vi "logging_stop.vi"(8 "error in":errorcluster caption="error in (no error)", 11 "VISA resource name":refnum<visa-resource-name>) -> (0 "error out":errorcluster, 3 "VISA resource name out":refnum<visa-resource-name>)   [LabVIEW 2020, in "Rohde&Schwarz RTx Oscilloscopes.lvlib" / "rsidr_core.lvlib"]
uses:
  rsidr_core.lvlib
  _type_Logging_Parameter.ctl
  type_Error_Codes.ctl
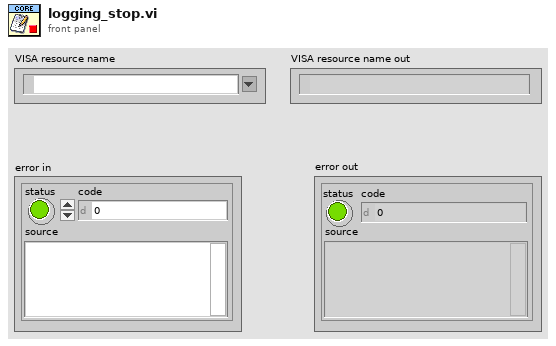
[diagram p1: front panel]
types:
  T1 = typedef "Rohde&Schwarz RTx Oscilloscopes.lvlib/rsidr_core.lvlib/_type_Logging_Parameter.ctl" = enum16{"Type (String)", "SessionAlias(String)", "FormatString (String)", "UDPconectionID (I32)", "UDPlocalPort (I32)", "UDPremotePort (I32)", "UDPremoteHost (String)", "FILEmode (I32)", "FILEpath (String)", "FILEopenID (I32)", "DataMaxLogLen (I32)"}
  T2 = typedef "Rohde&Schwarz RTx Oscilloscopes.lvlib/rsidr_core.lvlib/type_Error_Codes.ctl" = enum16{"No_error", "VISA_err_ResourceNotFound", "VISA_err_Timeout", "VISA_warn_MoreDataAvailable", "RS_err_MissingCallback", "RS_err_InvalidAttribute", "RS_err_InvalidValue", "RS_err_UnknownResource", "RS_err_AlreadyInitialized", "RS_err_InstrumentStatus", "RS_err_BadRepCapName", "RS_err_TypesMismatch", "RS_err_ValueNotSupported", "RS_err_InvalidRngTable", "RS_err_IDqueryFail", "RS_err_UnexpResponse", "VISA_warn_ConfigNotLoaded", "RS_err_AttributeNotReadable", "RS_err_AttributeNotWritable", "RS_err_InstrumentType", "RS_err_InstrumentOption", "VISA_err_InvalidSize", "RS_err_ReliabilityIndicator", "VISA_warn_UnknownStatus", "VISA_warn_TermCharRead", "VISA_err_IO_error", "RS_err_FunctionNotSupported", "VISA_warn_QueueEmpty"}
  T3 = typedef "Rohde&Schwarz RTx Oscilloscopes.lvlib/rsidr_core.lvlib/type_Session_Data.ctl" = cluster{"IDN string":string, "Instrument FW":string, "Instr type":string, "Instr type for err. msg.":string, "Installed Options":string[], "Ignore Error Messages":string, "Logging params":variant, "OPC Timeout":i32, "VISA Timeout":i32, "STB Poll VISA Timeout":i32, "Additional Flags":i32, "Wait Before Read":i32, "Wait Before Write":i32, "Option String Flags":i32, "IO Segment Size":i64, "VISA Access Mode":T4, "Interface Type":T5, "OPC Wait Mode":T6, "Bin Float Number  Format":T7, "Bin Integer Number Format":T8, "Simulate":bool, "VXIcapable":bool, "Duplicate Session":bool, "Add LF to Write":bool, "Logging":bool, "Fast Sweep":bool, "Query Instrument Status":bool, "Check Range":bool, "Check Options":bool, "OPC-sync Attr Writes":bool, "OPC-sync Attr Queries":bool}
  T4 = typedef "Rohde&Schwarz RTx Oscilloscopes.lvlib/rsidr_core.lvlib/type_VisaAccessMode.ctl" = u16
  T5 = typedef "Rohde&Schwarz RTx Oscilloscopes.lvlib/rsidr_core.lvlib/type_InterfaceType.ctl" = enum16{"Unknown", "GPIB", "VXI", "GPIB_VXI", "ASRL", "PXI", "TCPIP", "USB", "SOCKET"}
  T6 = typedef "Rohde&Schwarz RTx Oscilloscopes.lvlib/rsidr_core.lvlib/type_OPC_Wait_Mode.ctl" = enum16{"STBpolling", "STBpollingSlow", "STBpollingSuperSlow", "ServiceRequest", "OPCquery"}
  T7 = typedef "Rohde&Schwarz RTx Oscilloscopes.lvlib/rsidr_core.lvlib/type_Binary_Float_Number_Format.ctl" = enum16{"Float_4_Bytes_Swapped", "Float_4_Bytes", "Double_8_Bytes_Swapped", "Double_8_Bytes"}
  T8 = typedef "Rohde&Schwarz RTx Oscilloscopes.lvlib/rsidr_core.lvlib/type_Binary_Integer_Number_Format.ctl" = enum16{"Int32_4_Bytes_Swapped", "Int32_4 Bytes", "Int16_2_Bytes_Swapped", "Int16_2_Bytes"}
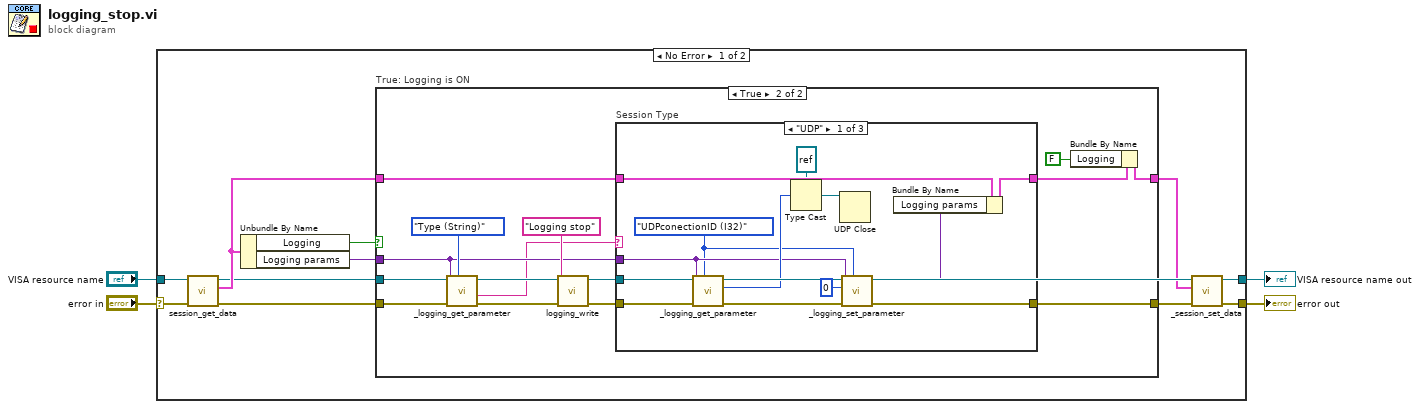
[diagram p0: block diagram]
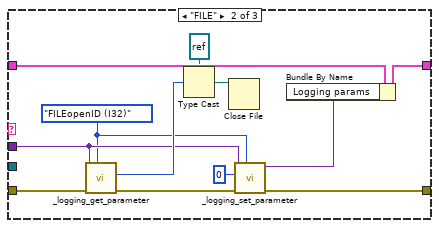
[diagram p3: hidden frame]
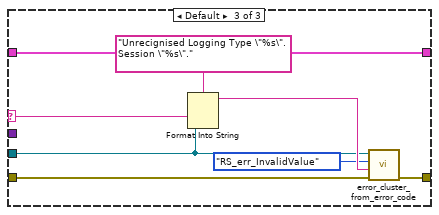
[diagram p4: hidden frame]
diagram:
  n1 = case shown="No Error" "error in" {
    selector: "error in" -> [w15 w65]
    tunnel: [w11 w65] -> w2
    tunnel: "VISA resource name" -> [w14 w64]
    tunnel: [w10 w64] -> w1
    frame No Error {
      n2 = call "session_get_data.vi"("error in"=w15, "VISA resource name"=w14) -> ("error out"=w13:errorcluster, "Session User Data out"=w8:T3, "VISA resource name out"=w7:refnum<visa-resource-name>)  [unwired: 6 in, 1 out]
      n3 = Unbundle By Name(w8) -> ("Logging"=w5:bool, "Logging params"=w9:variant)
      n4 = case "True: Logging is ON" shown="True" w5 {
        tunnel: w13 -> [w17 w22]
        tunnel: [w17 w31] -> w12
        tunnel: w9 -> [_ w20]
        tunnel: w8 -> [w16 w30]
        tunnel: [w16 w18] -> w6
        tunnel: w7 -> [_ w26]
        frame False {
        }
        frame True {
          n5 = call "_logging_get_parameter.vi"("Logging Parameter"=_type_Logging_Parameter."Type (String)", "error in"=w22, "Logging params in"=w20) -> ("error out"=w21:errorcluster, "String parameter out"=w19:string)  [unwired: 4 in, 3 out]
          n6 = call "logging_write.vi"("error in"=w21, "String to write"="Logging stop", "VISA resource name"=w26) -> ("error out"=w25:errorcluster, "VISA resource name out"=w24:refnum<visa-resource-name>)  [unwired: 7 in]
          n7 = case "Session Type" shown="\"UDP\"" w19 {
            selector: w19 -> [_ _ w63]
            tunnel: w25 -> [w41 w53 w61]
            tunnel: [w32 w46 w60] -> w31
            tunnel: w20 -> [w36 w50 _]
            tunnel: w30 -> [w42 w54 w59]
            tunnel: [w43 w55 w59] -> w28
            tunnel: w24 -> [_ _ w57]
            frame "UDP" {
              w33 = _type_Logging_Parameter."UDPconectionID (I32)" ("Logging Parameter")
              n8 = call "_logging_get_parameter.vi"("Logging Parameter"=w33, "error in"=w41, "Logging params in"=w36) -> ("error out"=w37:errorcluster, "Int32 parameter out"=w40:i32)  [unwired: 4 in, 3 out]
              n9 = Type Cast(type=refnum<k16> refnum ("connection ID"), x=w40) -> (*(type *) &x=w38:refnum<k16>)
              n10 = UDP Close(connection ID=w38) -> ()  [unwired: 1 in, 2 out]
              n11 = call "_logging_set_parameter.vi"("Logging Parameter"=w33, "error in"=w37, "Int32 parameter (0)"=0 ("I32 parameter (0)"), "Logging params in"=w36) -> ("error out"=w32:errorcluster, "Logging params out"=w35:variant)  [unwired: 6 in]
              n12 = Bundle By Name(cluster=w42, "Logging params"=w35) -> (w43:T3)
            }
            frame "FILE" {
              w47 = _type_Logging_Parameter."FILEopenID (I32)" ("Logging Parameter")
              n13 = call "_logging_get_parameter.vi"("Logging Parameter"=w47, "error in"=w53, "Logging params in"=w50) -> ("error out"=w51:errorcluster, "Int32 parameter out"=w52:i32)  [unwired: 4 in, 3 out]
              n14 = Type Cast(type=refnum<file> refnum ("refnum"), x=w52) -> (*(type *) &x=w44:refnum<file>)
              n15 = Close File(refnum=w44) -> ()  [unwired: 1 in, 2 out]
              n16 = call "_logging_set_parameter.vi"("Logging Parameter"=w47, "error in"=w51, "Int32 parameter (0)"=0 ("I32 parameter (0)"), "Logging params in"=w50) -> ("error out"=w46:errorcluster, "Logging params out"=w49:variant)  [unwired: 6 in]
              n17 = Bundle By Name(cluster=w54, "Logging params"=w49) -> (w55:T3)
            }
            frame Default {
              n18 = Format Into String(format string="Unrecignised Logging Type \"%s\". Session \"%s\".", w63, w57) -> (resulting string=w58:string)  [unwired: 2 in, 1 out]
              n19 = call "error_cluster_from_error_code.vi"("error in"=w61, "Error Message (\"\")"=w58, "Error Enum in"=type_Error_Codes."RS_err_InvalidValue", "VISA resource name"=w57) -> ("error out"=w60:errorcluster)  [unwired: 6 in, 1 out]
            }
          }
          n20 = Bundle By Name(cluster=w28, "Logging"=FALSE) -> (w18:T3)
        }
      }
      n21 = call "_session_set_data.vi"("error in"=w12, "Session User Data in"=w6, "VISA resource name"=w7) -> ("error out"=w11:errorcluster, "VISA resource name out"=w10:refnum<visa-resource-name>)  [unwired: 7 in]
    }
    frame Error {
    }
  }
  "VISA resource name out" <- w1
  "error out" <- w2
